vi "Copy Value.vi"(8 "error in (no error)":errorcluster, 10 "From":refnum<class "Type.lvclass">, 11 "Boolean in":refnum<class "Boolean.lvclass">) -> (0 "error out":errorcluster, 3 "Boolean out":refnum<class "Boolean.lvclass">)   [LabVIEW 2022 SP3, in "Conditum.lvlib" / "Columns.lvlib" / "Boolean.lvclass"]
uses:
  Boolean.lvclass
  Boolean.lvclass/Boolean.ctl
  Type/Type.lvclass
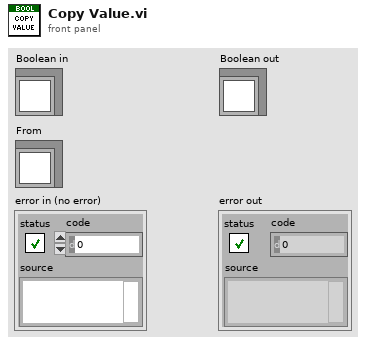
[diagram p1: front panel]
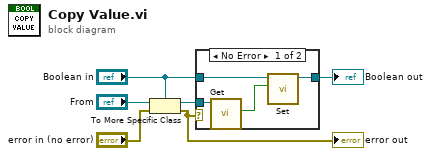
[diagram p0: block diagram]
diagram:
  n1 = To More Specific Class(target class="Boolean in", reference="From", error in="error in (no error)") -> (specific class reference=w4:refnum<class "Boolean.lvclass">, error out=w1:errorcluster)
  "error out" <- w1
  n2 = case shown="No Error" w1 {
    tunnel: w4 -> [w10 _]
    tunnel: "Boolean in" -> [w8 w11]
    tunnel: [w7 w11] -> w2
    frame No Error {
      n3 = call "Get.vi"("Boolean in"=w10) -> ("Value"=w9:bool)  [unwired: 10 in]
      n4 = call "Set.vi"("Value"=w9, "Boolean in"=w8) -> ("Boolean out"=w7:refnum<class "Boolean.lvclass">)  [unwired: 9 in]
    }
    frame Error {
    }
  }
  "Boolean out" <- w2
